vi "Utilization Heartbeat HTTP.vi"(8 "error in (no error)":errorcluster, 10 "configuration":refnum<class "NI Skyline Configuration HTTP.lvclass">, 11 "utilizationIdentifier":string) -> (0 "error out":errorcluster)   [LabVIEW 2023, in "Logger.lvclass"]
uses:
  Logger.lvclass
  <vilib>/Skyline/Configuration/Configuration HTTP_class/NI Skyline Configuration HTTP.lvclass
  <vilib>/Skyline/Configuration/Configuration HTTP_class/NI Skyline Configuration HTTP.lvclass/NI Skyline Configuration HTTP.ctl
  <vilib>/Skyline/Configuration/Configuration HTTP_class/Read Server URL.vi
  <vilib>/httpClient/POSTBuffer.vi
  <vilib>/httpClient/LabVIEWHTTPClient.lvlib
panel:
  out "URL":string
  out "JSON string":string
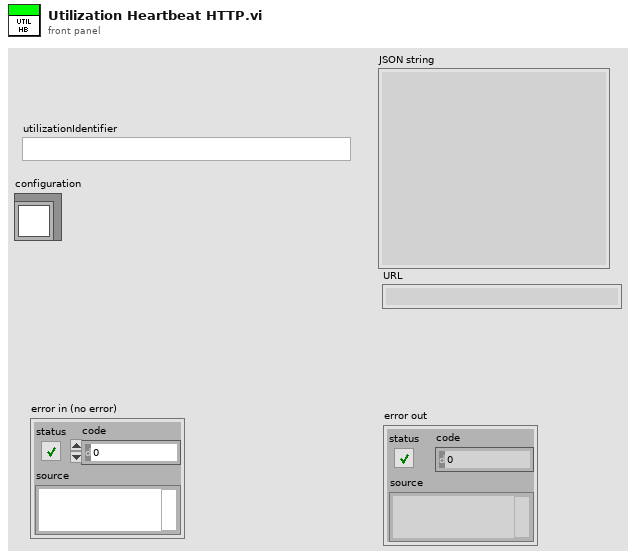
[diagram p1: front panel]
types:
  T1 = cluster{"utilizationIdentifiers":string[], "utilizationTimestamp":string}
  T2 = typedef "LabVIEWHTTPClient.lvlib/ClientHandle.ctl" = refnum<k1>
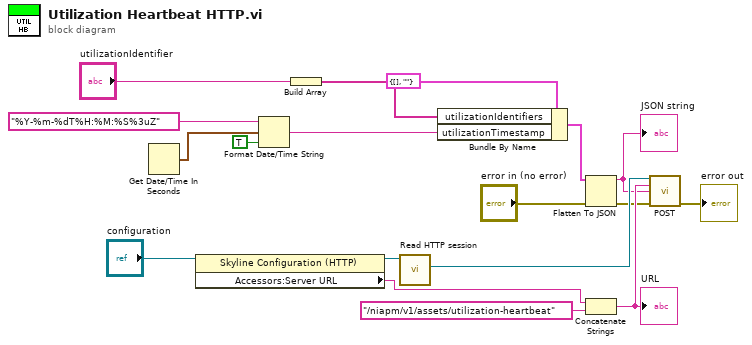
[diagram p0: block diagram]
diagram:
  n1 = Get Date/Time In Seconds() -> (seconds since 1Jan1904=w15:timestamp)
  n2 = property class="Skyline Configuration (HTTP)"(reference="configuration") -> (reference out=w11:refnum<class "NI Skyline Configuration HTTP.lvclass">, "Accessors:Server URL"=w9:string)  [unwired: 1 in, 1 out]
  n3 = Format Date/Time String(time format string (%c)="%Y-%m-%dT%H:%M:%S%3uZ", seconds (now)=w15, UTC format=TRUE) -> (date/time string=w18:string)
  n4 = Build Array("utilizationIdentifier") -> (w1:string[])
  n5 = call <vilib>:"Read HTTP session.vi"("HTTP configuration in"=w11) -> ("http session"=w10:T2)  [unwired: 8 in, 2 out]
  n6 = Bundle By Name(cluster=T1 {"utilizationIdentifiers"=[], "utilizationTimestamp"=""}, "utilizationIdentifiers"=w1, "utilizationTimestamp"=w18) -> (w14:T1)
  n7 = Flatten To JSON(anything=w14, error in (no error)="error in (no error)") -> (JSON string=w6:string, 11:w5:errorcluster)  [unwired: 1 in]
  "JSON string" <- w6
  n8 = Concatenate Strings(w9, "/niapm/v1/assets/utilization-heartbeat") -> (w7:string)
  "URL" <- w7
  n9 = call-poly <vilib>:"POST.vi"("client handle"=w10, "url"=w7, "buffer"=w6, "error in (no error)"=w5) -> ("error out"=→"error out":errorcluster)  [unwired: 8 in, 3 out]
